vi "Agilis cfg Ch1Ax2Pos.vi"(8 "error in (no error)":errorcluster, 9 "Channel parsed command info":T1, 10 "Simulation":T2, 11 "input cluster":refnum<class "AgilisPiezoStage.lvclass">) -> (0 "error out":errorcluster, 1 "new commands":string, 3 "output cluster":refnum<class "AgilisPiezoStage.lvclass">)   [LabVIEW 2013, in "AgilisPiezoStage.lvclass"]
uses:
  AgilisPiezoStage.lvclass
  shared/OnOffTypeDef.ctl
  Shared/Device Driver/channel parsed cmd cluster.ctl
  AgilisPiezoStage.lvclass/AgilisPiezoStage.ctl
  C:/Program Files/Newport/Piezo Motion Control/Newport AG-UC2-UC8 Applet/Samples/LabVIEW 2009/AgilisCmdLib.dll
  Program Files/Newport/Piezo Motion Control/Newport AG-UC2-UC8 Applet/Samples/LabVIEW 2009/AgilisCmdLib.dll
  shared/CompressAndUpdate(Poly)/CompressAndUpdate(Numeric).vi
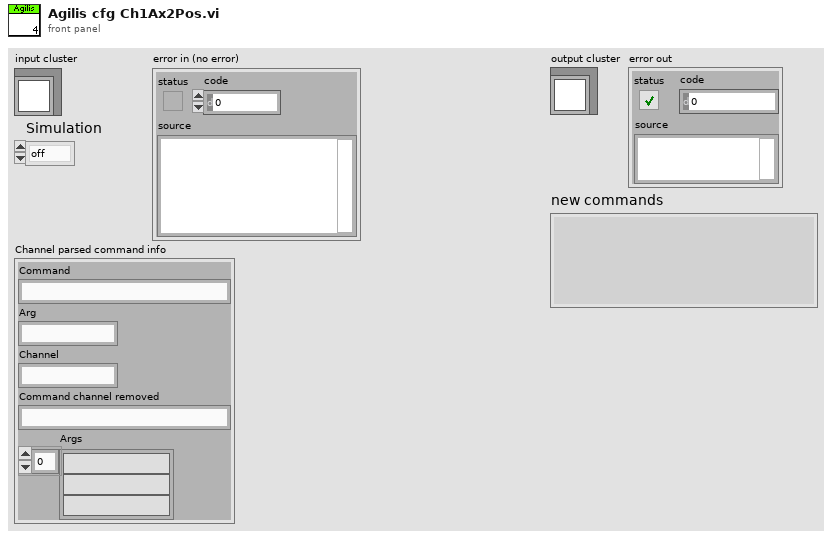
[diagram p1: front panel]
types:
  T1 = typedef "channel parsed cmd cluster.ctl" = cluster{"Command":string, "Arg":string, "Channel":string, "Command channel removed":string, "Args":string[]}
  T2 = typedef "OnOffTypeDef.ctl" = enum16{"off", "on"}
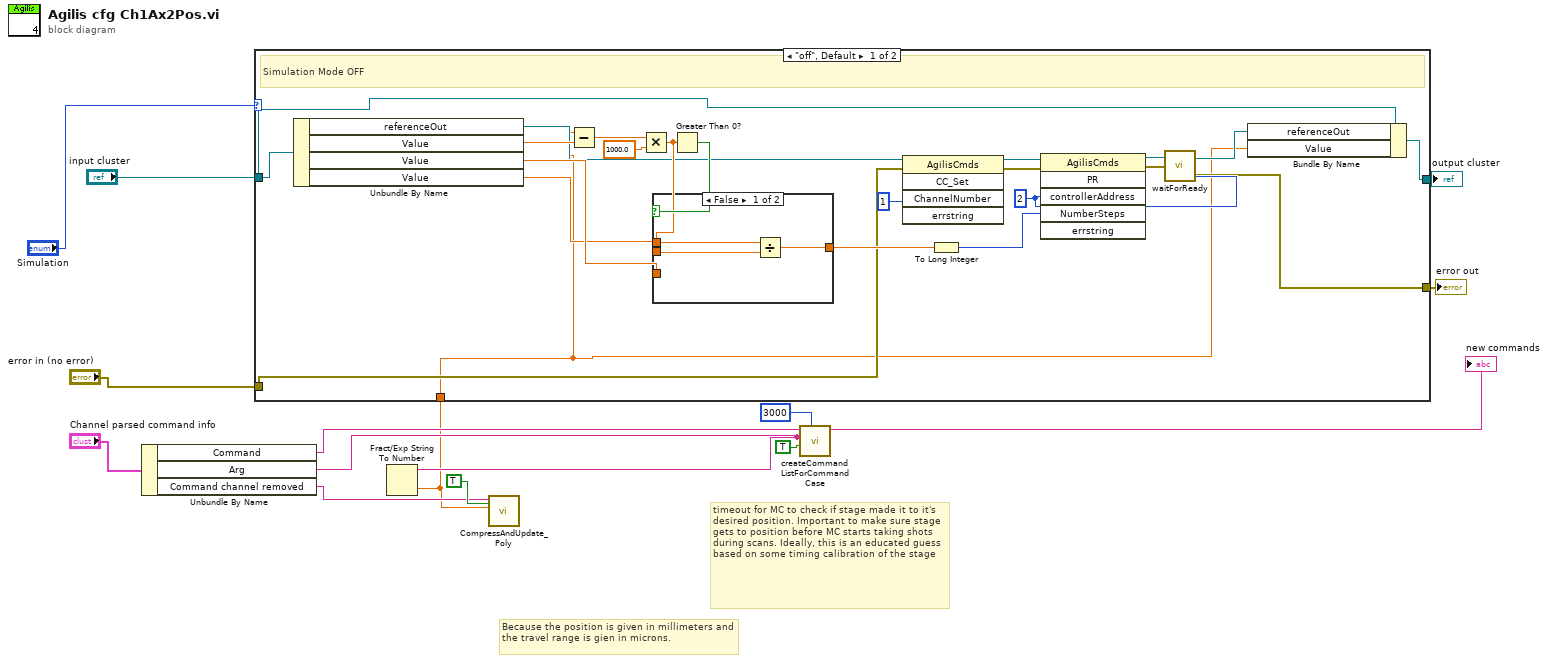
[diagram p0: block diagram]
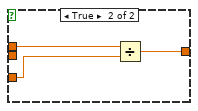
[diagram p2: hidden frame]
diagram:
  # "timeout for MC to check if stage made it to it's desired position. Important to make sure stage gets to position before MC starts taking shots during scans. Ideally, this is an educated guess based on some timing calibration of the stage"
  # "Because the position is given in millimeters and the travel range is gien in microns."
  n1 = Unbundle By Name("Channel parsed command info") -> ("Command"=w11:string, "Arg"=w10:string, "Command channel removed"=w9:string)
  n2 = Fract/Exp String To Number(string=w10) -> (number=w2:dbl)  [unwired: 3 in, 1 out]
  n3 = case shown="\"off\", Default" "Simulation" {
    tunnel: [w36 w44] -> w5
    tunnel: "input cluster" -> [w35 w44]
    tunnel: "error in (no error)" -> [w22 w43]
    tunnel: [w16 w43] -> w4
    tunnel: w2 -> [w15 _]
    frame "off", Default {
      w20 = 2 ("controllerAddress")
      # "Simulation Mode OFF"
      n4 = Unbundle By Name(w35) -> ("referenceOut"=w24:refnum<k24>, "Value"=w32:dbl, "Value"=w27:dbl, "Value"=w26:dbl)
      n5 = Subtract(x=w15, y=w32) -> (x-y=w34:dbl)
      n6 = Multiply(x=w34, y=1000.0) -> (x*y=w28:dbl)
      n7 = Greater Than 0?(x=w28) -> (x > 0?=w31:bool)
      n8 = case shown="False" w31 {
        tunnel: w28 -> [w39 w42]
        tunnel: [w38 w41] -> w30
        tunnel: w27 -> [_ w40]
        tunnel: w26 -> [w37 _]
        frame False {
          n9 = Divide(x=w39, y=w37) -> (x/y=w38:dbl)
        }
        frame True {
          n10 = Divide(x=w42, y=w40) -> (x/y=w41:dbl)
        }
      }
      n11 = invoke class="AgilisCmds" method="CC_Set"(reference=w24, error in=w22, "ChannelNumber"=1) -> (reference out=w23:refnum<k24>, error out=w21:errorcluster)  [unwired: 2 in, 3 out]
      n12 = To Long Integer(number=w30) -> (32bit integer=w29:i32)
      n13 = invoke class="AgilisCmds" method="PR"(reference=w23, error in=w21, "controllerAddress"=w20, "NumberSteps"=w29) -> (reference out=w19:refnum<k24>, error out=w18:errorcluster)  [unwired: 2 in, 4 out]
      n14 = call "waitForReady.vi"("axis"=w20, "errorIn"=w18, "referenceIn"=w19) -> ("errorOut"=w16:errorcluster, "referenceOut"=w17:refnum<k24>)
      n15 = Bundle By Name(cluster=w35, "referenceOut"=w17, "Value"=w15) -> (w36:refnum<class "AgilisPiezoStage.lvclass">)
    }
    frame "on" {
      # "Simulation Mode ON"
    }
  }
  "output cluster" <- w5
  "error out" <- w4
  n16 = call-poly "CompressAndUpdate_Poly.vi"("force CVT update (false)"=TRUE ("force CVT update"), "Numeric"=w2, "command or variable name"=w9) -> ()  [unwired: 8 in, 1 out]
  n17 = call "createCommandListForCommandCase.vi"("timeout (optional)"=3000, "immediate Check (only once)"=TRUE, "setvalue"=w10, "command"=w11) -> ("new commands"=→"new commands":string)  [unwired: 7 in]
